vi "Dust_Control_Giraffe_small.vi"(7 "error in":errorcluster) -> (0 "error out":errorcluster)   [LabVIEW 2013]
doc: "This VI specifies the properties of the pulse used for running the dust source. When program is stopped, the voltage is incrementally reduced to zero to avoid quick drops."
uses:
  <vilib>/Utility/miscctls.llb/LVPointTypeDef.ctl
  Functional Global Variables/Action Items.ctl
  <vilib>/Utility/error.llb/DialogType.ctl
  <vilib>/DAQmx/read.llb/DAQmx Read (Analog 1D Wfm NChan NSamp).vi
  <vilib>/Analysis/baseanly.llb/Mean (DBL).vi
  <vilib>/DAQmx/write.llb/DAQmx Write (Analog 1D Wfm NChan NSamp).vi
  <vilib>/DAQmx/read.llb/DAQmx Read (Counter U32 1Chan 1Samp).vi
  <vilib>/addons/database/Connection.llb/Conn Execute.vi
  <vilib>/addons/database/Recordset.llb/Rec Fetch Recordset Data (R).vi
  <vilib>/addons/database/Recordset.llb/Rec Destroy - Connection.vi
  <vilib>/DAQmx/create/channels.llb/DAQmx Create Channel (AI-Voltage-Basic).vi
  <vilib>/DAQmx/configure/timing.llb/DAQmx Timing (Sample Clock).vi
  <vilib>/DAQmx/create/channels.llb/DAQmx Create Channel (AO-Voltage-Basic).vi
  <vilib>/DAQmx/create/channels.llb/DAQmx Create Channel (CI-Count Edges).vi
  <userlib>/_OpenG.lib/comparison/comparison.llb/DBL Changed__ogtk.vi
  <vilib>/measure/mascope.llb/Amplitude and Levels 1 chan.vi
  <vilib>/DAQmx/miscellaneous.llb/DAQmx Fill In Error Info.vi
  Private/throttle.vi
  <userlib>/_OpenG.lib/comparison/comparison.llb/Boolean Changed__ogtk.vi
  Private/throttle from query.vi
  <vilib>/addons/database/_DB Variant To Data/Database Variant To Data.xnode
  <resource>/objmgr/daqmx.rc
  <vilib>/measure/NI_MAPro.lvlib
  <vilib>/Analysis/NI_AALBase.lvlib
  <vilib>/addons/database/NI_Database_API.lvlib
panel:
  out "Freq. Before Throttle":dbl
  out "On/Off":bool
  out "Finished":bool=TRUE
  out "Output waveform":waveform(dbl)={"t0"=timestamp(0 s since 1904-01-01), "dt"=4e-06, "Y"=array[50000 elements]}
  out "Input waveform":waveform(dbl)={"t0"=timestamp(3437998856.0330505 s since 1904-01-01), "dt"=0.00019999999999999998, "Y"=array[1000 elements], "attributes"=variant("NI_ChannelName"=variant(string "Dev5/ai20"), "NI_UnitDescription"=variant(string "Volts"))}
  out "output cluster":T1={"Integer Timestamp"=0, "Needle Voltage"=0.0, "Frequency"=1.0, "Width (ms) : 0.1 "=0.1, "Desired Amplitude (V)"=0.0, "Settings ID"="", "ID#"=0} {"Needle Voltage" min=0.0 max=10.0 step=0.01 format="%.2g"; "Desired Amplitude (V)" min=0.0 max=10.0 step=0.01 format="%5.2f"; "Width (ms) : 0.1" min=0.05 max=5.0 step=0.01 format="%6.2f"; "Frequency" min=1.0 max=100.0 step=0.01 format="%.1f"}
  in  "Tab Control":enum32{"Controls", "Status", "Counter"}(tab)
  in  "Big Accelerator\nSetting?":bool
  out "Actual output width (ms)":dbl caption="Actual Output Width (ms)" format="%.2f"
  out "Actual output Frequency":dbl caption="Actual Output  Frequency (hz)" format="%.2f"
  in  "Width (ms) : 0.1":dbl=0.1 min=0.0 max=5.0 step=0.01 format="%6.2f"
  out "Actual Amplitude (V) 2":dbl=0.0012999050305587314 caption="Actual Amplitude (V)" format="%.2f"
  in  "Desired Amplitude (V)":dbl min=0.0 max=10.0 step=0.01 format="%5.2f"
  out "Actual output Amplitude (V)":dbl caption="Actual Output Amplitude (V)" format="%.2f"
  in  "Frequency":dbl=1.0 caption="Frequency (Hz) : 1" min=0.0 max=30.0 step=0.01 format="%.1f"
  in  "Abort Change":bool
  out "Actual Needle (kV)":dbl=-1.1093266413053247 caption="Actual Einzel (V)" format="%.2f"
  out "Actual Needle Output (V)":dbl caption="Actual Einzel (V)" format="%.2f"
  in  "Needle Voltage":dbl min=0.0 max=10.0 step=0.01 format="%.2g"
  in  "Save Settings?":bool
  out "CONTROLS":waveform(dbl)[](graph)=[{"t0"=timestamp(0 s since 1904-01-01), "dt"=4e-06, "Y"=array[50000 elements]}, {"t0"=timestamp(3437998856.0330505 s since 1904-01-01), "dt"=0.00019999999999999998, "Y"=array[1000 elements], "attributes"=variant("NI_ChannelName"=variant(string "Dev5/ai20"), "NI_UnitDescription"=variant(string "Volts"))}]
  in  "Settings ID":string
  in  "Retrieve Settings":bool
  out "Ratio of particles at\nsecond detector to first":dbl
  out "First detector since\nlast source change:":i64
  out "Average Rate of first":dbl
  out "Average Rate of second":dbl
  in  "# of Cycles ot Average":i32=10
  out "Number of Hours":dbl
  out "Chamber Pressure":dbl format="%#_3g"
  in  "Physical Channels":tag="Dev4/ao0:1" caption="Physical Output Channels"
  in  "Physical Input Channels":tag="Dev6/ai0:2"
  out "Execution Number:":i32=341
  out "Testing":bool
  in  "Counters On/Off":bool=TRUE
  in  "Reset Counters":bool
  in  "Det1":tag="Dev5/ctr0"
  in  "Det2":tag="Dev5/ctr1"
  out "Det2":u32
  out "Det1":u32
  out "error?":bool
  out "Actual Sample Clock Rate":dbl=250000.0 format="%.2f"
  in  "stop":bool
  # "CCLDAS Dust Control Small Accelerator"
  # "Hold Down to\nStop Changes"
  # "Tube Drive (Ao0, Ai4)"
  # "Needle Control (Ao4, Ai0)"
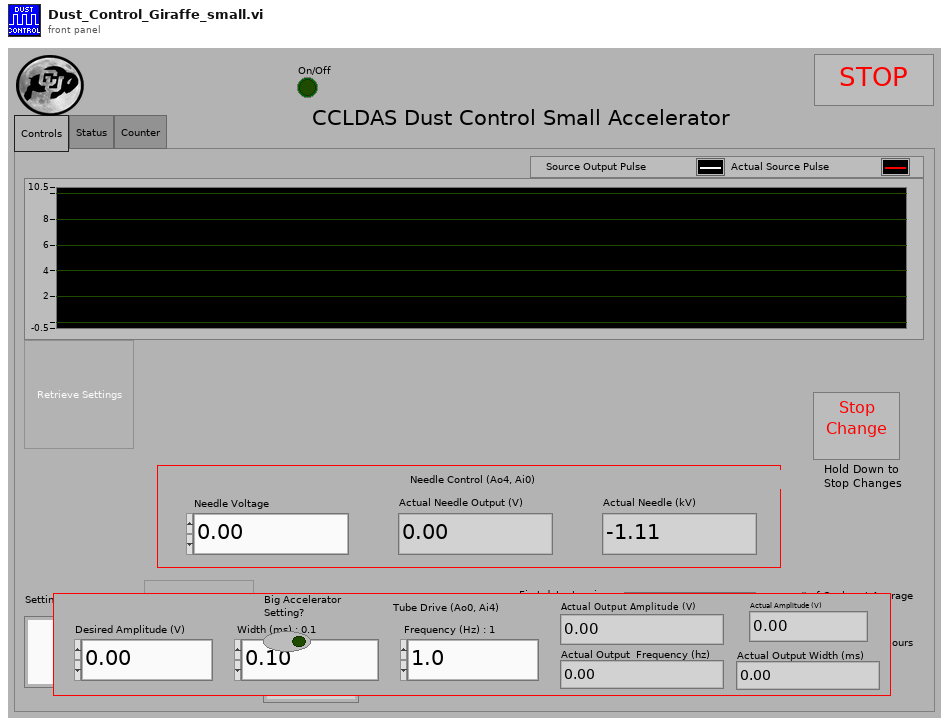
[diagram p1: front panel]
types:
  T1 = cluster{"Integer Timestamp":u64, "Needle Voltage":dbl, "Frequency":dbl, "Width (ms) : 0.1 ":dbl, "Desired Amplitude (V)":dbl, "Settings ID":string, "ID#":i32}
  T2 = typedef "Action Items.ctl" = enum16{"Initialize", "Get", "Set"}
  T3 = typedef "LVPointTypeDef.ctl" = cluster{"Horizontal":i16, "Vertical":i16}
  T4 = typedef "NI_Database_API.lvlib/Conn ObjectReference.ctl" = refnum<k1>
  T5 = typedef "NI_Database_API.lvlib/Rec ObjectReference.ctl" = refnum<k1>
  T6 = enum8{"Enabled", "Disabled", "Disabled and Grayed Out"}
  T7 = typedef "DialogType.ctl" = u16
  T8 = cluster{"Integer Time":i64, "Integer Time":i64, "data":i32}
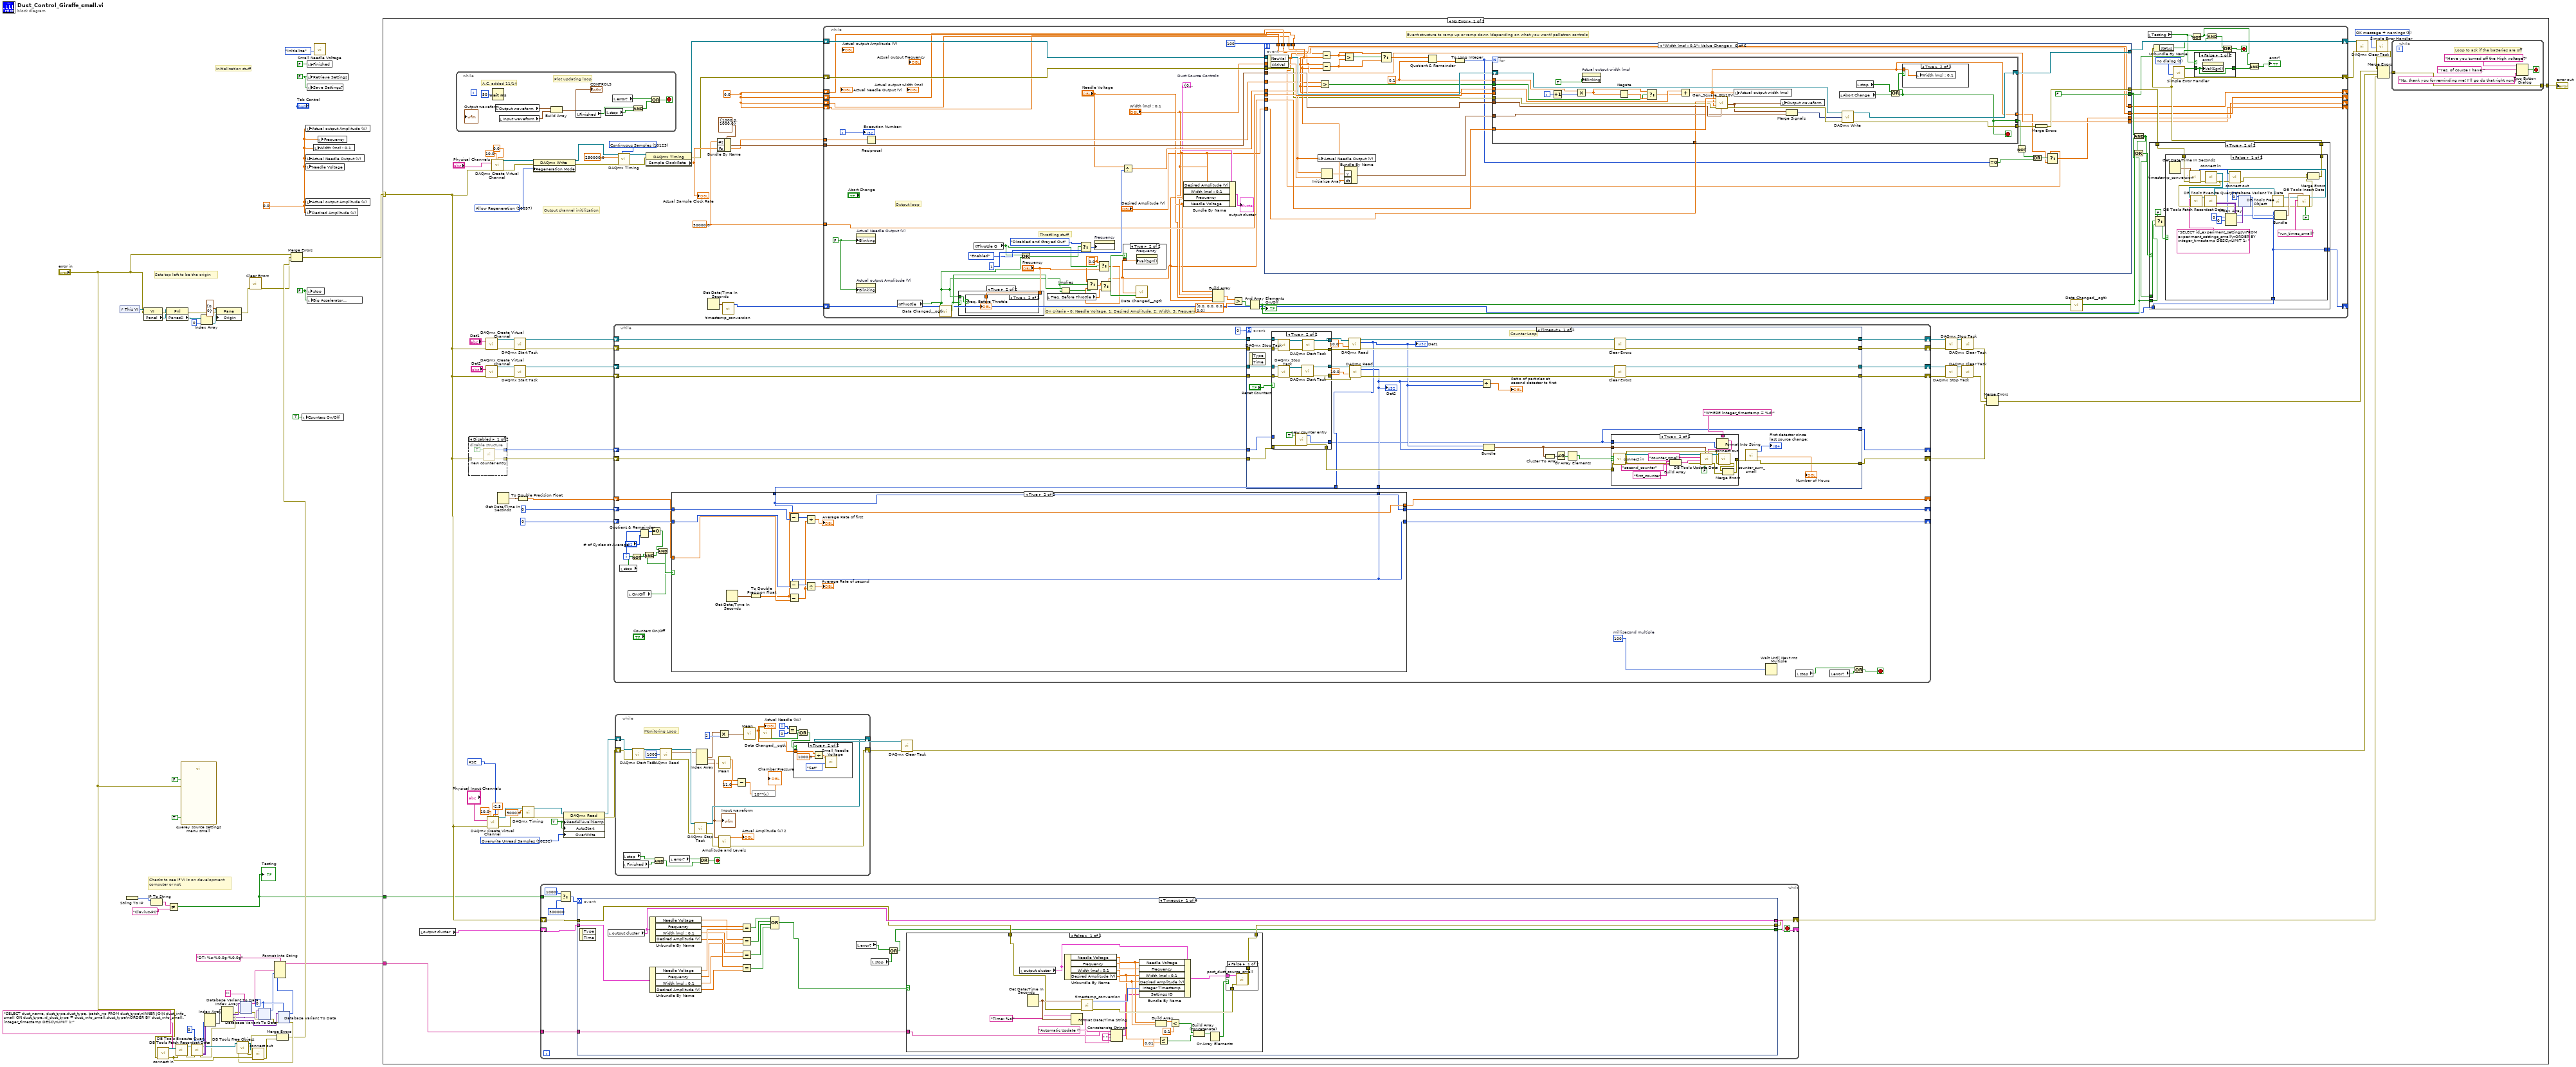
[diagram p0: block diagram]
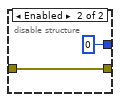
[diagram p2: hidden frame]
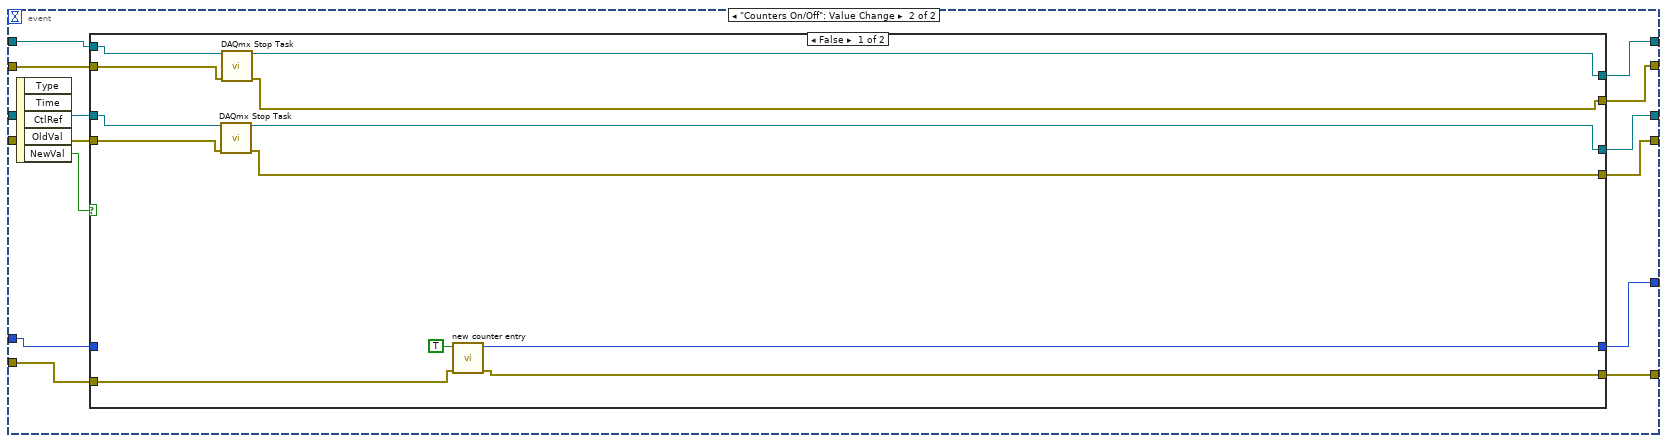
[diagram p5: hidden frame]
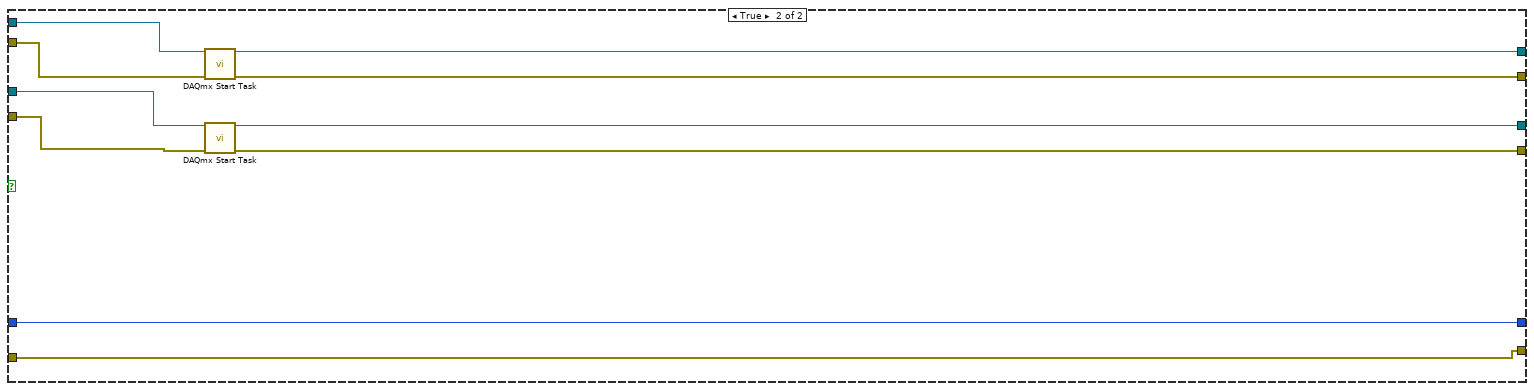
[diagram p6: hidden frame]
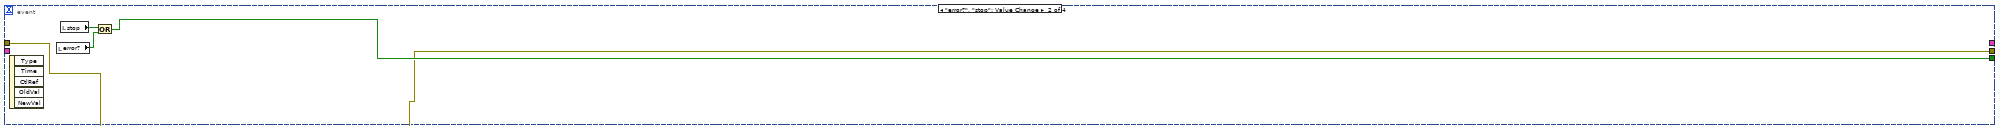
[diagram p11: hidden frame]
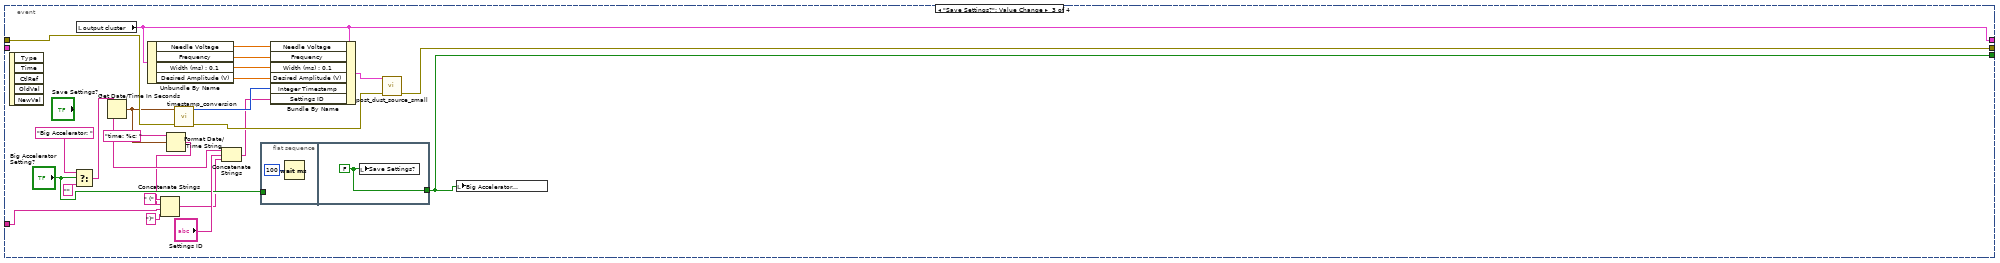
[diagram p12: hidden frame]
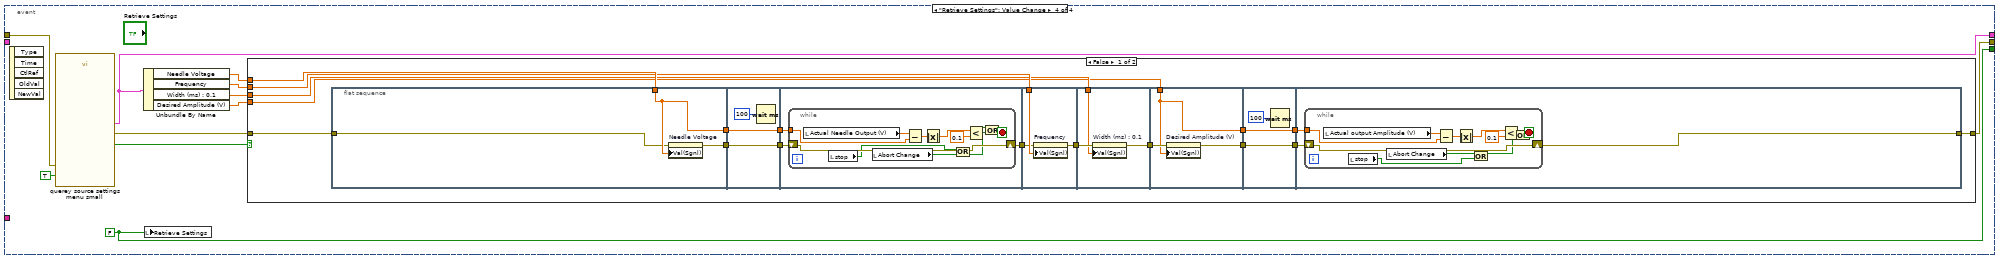
[diagram p13: hidden frame]
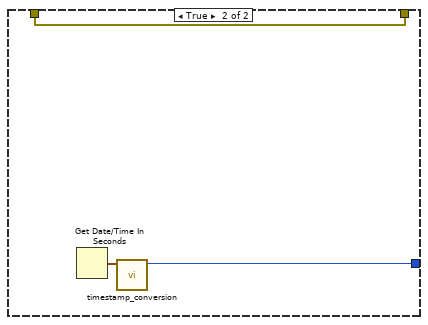
[diagram p19: hidden frame]
diagram:
  w15 = 0
  w50 = FALSE ("Retrieve Settings")
  w48 = 0.0 ("Actual Output (V)")
  w47 = FALSE ("Shutdown")
  # "Checks to see if VI is on development\ncomputer or not"
  # "Sets top left to be the origin"
  # "Initialization stuff"
  n1 = control-ref of="This VI"() -> (w46:refnum<vi>)
  n2 = String To IP() -> (0:w38:u32)  [unwired: 1 in]
  n3 = property class="VI"(reference=w46, error in="error in") -> (error out=w45:errorcluster, "Panel"=w44:refnum<vi>)  [unwired: 1 out]
  n4 = IP To String(2:w38) -> (0:w37:string)  [unwired: 1 in]
  n5 = call "connect in.vi"("error in (no error)"="error in") -> ("error out"=w32:errorcluster, "Database Connection"=w35:T4)  [unwired: 6 in, 1 out]
  n6 = property class="Pnl"(reference=w44, error in=w45) -> (error out=w43:errorcluster, "Panes[]"=w42:refnum<vi>[])  [unwired: 1 out]
  n7 = Not Equal?(x=w37, y="Clavius-PC") -> (x != y?=w8:bool)
  "Testing" <- w8
  n8 = call-poly <vilib>:"DB Tools Execute Query.vi"("error in (no error)"=w32, "SQL query"="SELECT dust_name, dust_type.dust_type, batch_no FROM dust_type\nINNER JOIN dust_info_small ON dust_type.id_dust_type = dust_info_small.dust_type\nORDER BY dust_info_small.integer_timestamp DESC\nLIMIT 1;", "connection reference"=w35) -> ("error out"=w34:errorcluster, "recordset reference"=w33:T5)  [unwired: 5 in]
  n9 = call "querey source settings menu small.vi"("Enable"=FALSE, "subvi?"=TRUE, "error in (no error)"="error in") -> ()  [unwired: 13 in, 4 out]
  n10 = call-poly <vilib>:"DB Tools Fetch Recordset Data.vi"("error in (no error)"=w34, "recordset reference"=w33) -> ("error out"=w20:errorcluster, "recordset data"=w30:variant[][], "recordset reference out"=w29:T5)  [unwired: 3 in]
  n11 = Index Array(array=w42, index=0) -> (element=w40:refnum<vi>)
  n12 = Index Array(array=w30, index (row)=0) -> (element=w24:variant[])  [unwired: 1 in]
  n13 = property class="Pane"(reference=w40, error in=w43, "Origin"=T3 {"Horizontal"=0, "Vertical"=0}) -> (error out=w3:errorcluster)  [unwired: 1 out]
  n14 = Index Array(array=w24) -> (element #1=w23:variant, element #2=w18:variant, element #3=w17:variant)  [unwired: 3 in]
  n15 = xnode "Database Variant To Data"("database variant"=w23, "error in (no error)"=w20, "type"="") -> ("data"=w13:string, "error out"=w22:errorcluster)
  n16 = call <vilib>:"Clear Errors.vi"("error in (no error)"=w3) -> ("error out"=w4:errorcluster)  [unwired: 6 in]
  n17 = xnode "Database Variant To Data"("database variant"=w18, "error in (no error)"=w22, "type"=w15) -> ("data"=w12:i32, "error out"=w21:errorcluster)
  n18 = xnode "Database Variant To Data"("database variant"=w17, "error in (no error)"=w21, "type"=w15) -> ("data"=w11:i32, "error out"=w19:errorcluster)
  n19 = call-poly <vilib>:"DB Tools Free Object.vi"("error in (no error)"=w19, "recordset reference"=w29) -> ("error out"=w28:errorcluster, "connection reference"=w25:T4)  [unwired: 8 in]
  n20 = call "connect out.vi"("error in (no error)"=w32, "connection reference"=w25) -> ("error out"=w27:errorcluster)  [unwired: 9 in]
  n21 = Format Into String(format string="DT: %s-%0.0g-%0.0g", w13, w12, w11) -> (resulting string=w9:string)  [unwired: 2 in, 1 out]
  n22 = Merge Errors(w28, w27) -> (w10:errorcluster)
  n23 = Merge Errors("error in", w4, w10) -> (w5:errorcluster)
  n24 = local write "Counters On/Off"(TRUE ("Counters On/Off")) -> ()
  n25 = local write "Actual output Amplitude (V)"(w48) -> ()
  n26 = local write "Actual Needle Output (V)"(w48) -> ()
  n27 = local write "Needle Voltage"(w48) -> ()
  n28 = local write "Actual output Amplitude (V)"(w48) -> ()
  n29 = local write "Desired Amplitude (V)"(w48) -> ()
  n30 = local write "Finished"(FALSE ("Finished")) -> ()
  n31 = local write "Retrieve Settings"(w50) -> ()
  n32 = local write "Save Settings?"(w50) -> ()
  n33 = local write "stop"(w47) -> ()
  n34 = local write "Big Accelerator\nSetting?"(w47) -> ()
  n35 = local write "Width (ms) : 0.1"(w48) -> ()
  n36 = call "Small Needle Voltage.vi"("Action"=Action_Items."Initialize") -> ()  [unwired: 10 in, 1 out]
  n37 = local write "Frequency"(w48) -> ()
  n38 = case shown="No Error" w5 {
    selector: w5 -> [w65 w994]
    tunnel: [w107 w994] -> w52
    tunnel: w9 -> [w55 _]
    tunnel: w8 -> [w54 _]
    frame No Error {
      w53 = 10083 items=["default"=-1, "RSE"=10083, "NRSE"=10078, "Differential"=10106, "Pseudodifferential"=12529] ("input terminal configuration")
      w62 = 0.0 ("Width (ms) : 3.5")
      w75 = 10252 items=["Overwrite Unread Samples"=10252, "Do Not Overwrite Unread Samples"=10159] ("OverWrite")
      w76 = TRUE ("ReadAllAvailSamp")
      w58 = 50000.0 ("Size (Samples)")
      w120 = 10097 items=["Allow Regeneration"=10097, "Do Not Allow Regeneration"=10158] ("RegenMode")
      w125 = T7 3 items=["no dialog", "OK message", "continue or stop message", "OK message + warnings", "continue/stop + warnings"] ("type of dialog (OK msg:1)")
      w129 = 10123 items=["Finite Samples"=10178, "Continuous Samples"=10123] ("sample mode")
      # "Output channel initilization"
      n39 = local read "output cluster"() -> (w57:T1)
      n40 = while {
        stop <- w304 stop-if-true
        # "Plot updating loop"
        # "A.C. added 11/14"
        n41 = Wait (ms)(milliseconds to wait=u32 50) -> ()  [unwired: 1 out]
        n42 = local read "Output waveform"() -> (w301:waveform(dbl))
        n43 = local read "Input waveform"() -> (w302:waveform(dbl))
        n44 = Build Array(w301, w302) -> (→"CONTROLS":waveform(dbl)[])
        n45 = local read "Finished"() -> (w299:bool)
        n46 = local read "stop"() -> (w300:bool)
        n47 = local read "error?"() -> (w303:bool)
        n48 = And(x=w299, y=w300) -> (x .and. y?=w298:bool)
        n49 = Or(x=w303, y=w298) -> (x .or. y?=w304:bool)
      }
      n50 = disable-structure shown="Disabled" {
        disable-tunnel: [w133 w135] -> w84
        disable-tunnel: [w132 i64 0 ("Integer Time")] -> w83
        disable-tunnel: w65 -> [w131 w135]
        frame Disabled {
          n51 = call "new counter entry.vi"("error in"=w131, "Small?"=TRUE) -> ("error out"=w133:errorcluster, "Integer Time"=w132:i64)  [unwired: 8 in]
        }
        frame Enabled {
        }
      }
      n52 = call-poly <vilib>:"DAQmx Create Virtual Channel.vi"("counter"="Det1", "error in"=w65) -> ("task out"=w92:refnum<k21>, "error out"=w89:errorcluster)  [unwired: 12 in]
      n53 = call-poly <vilib>:"DAQmx Create Virtual Channel.vi"("counter"="Det2", "error in"=w65) -> ("task out"=w91:refnum<k21>, "error out"=w90:errorcluster)  [unwired: 12 in]
      n54 = call-poly <vilib>:"DAQmx Create Virtual Channel.vi"("maximum value"=10.0 ("Maximum Value"), "minimum value"=-2.5 ("Minimum Value"), "input terminal configuration"=w53, "physical channels"="Physical Input Channels", "error in"=w65) -> ("task out"=w69:refnum<k21>, "error out"=w68:errorcluster)  [unwired: 9 in]
      n55 = call-poly <vilib>:"DAQmx Create Virtual Channel.vi"("maximum value"=10.0 ("Maximum Value"), "minimum value"=0.0 ("Minimum Value"), "physical channels"="Physical Channels", "error in"=w65) -> ("task out"=w119:refnum<k21>, "error out"=w118:errorcluster)  [unwired: 10 in]
      n56 = Get Date/Time In Seconds() -> (seconds since 1Jan1904=w82:timestamp)
      n57 = call <vilib>:"DAQmx Start Task.vi"("task/channels in"=w92, "error in"=w89) -> ("task out"=w104:refnum<k21>, "error out"=w101:errorcluster)  [unwired: 12 in]
      n58 = call <vilib>:"DAQmx Start Task.vi"("task/channels in"=w91, "error in"=w90) -> ("task out"=w103:refnum<k21>, "error out"=w102:errorcluster)  [unwired: 12 in]
      n59 = To Double Precision Float(number=w82) -> (double precision float=w81:dbl)
      n60 = call-poly <vilib>:"DAQmx Timing.vi"("task/channels in"=w69, "rate"=5000.0, "error in"=w68) -> ("task out"=w74:refnum<k21>, "error out"=w73:errorcluster)  [unwired: 11 in]
      n61 = property class="DAQmx Write"(reference=w119, error in=w118, "Regeneration Mode"=w120) -> (reference out=w117:refnum<k21>, error out=w116:errorcluster)
      n62 = while {
        shift-right: [w349] -> w86
        shift-left: w65 -> [w348]
        shift-right: [w351] -> _
        shift-left: w57 -> [w350]
        tunnel: w54 -> [w344]
        tunnel: w55 -> [w342]
        stop <- w347 stop-if-true
        n63 = Select(t=1000, s=w344, f=300000) -> (s? t:f=w346:i32)
        n64 = event shown="[0] Timeout" {
          selector: _ -> [_ _ _ _]
          dyn-events: _ -> [_ _ _ _]
          timeout: w346 -> [_ _ _ _]
          tunnel: [w372 _ w414 w433] -> w351
          tunnel: w350 -> [w371 _ _ _]
          tunnel: [w356 w402 w429 w436] -> w349
          tunnel: w348 -> [w357 w402 w426 w442]
          tunnel: [w354 w403 w415 w435] -> w347
          tunnel: w342 -> [w358 _ w410 _]
          event Timeout {
            n65 = event-data() -> ()  [unwired: 1 in, 2 out]
            n66 = local read "output cluster"() -> (w372:T1)
            n67 = Unbundle By Name(w372) -> ("Needle Voltage"=w370:dbl, "Frequency"=w368:dbl, "Width (ms) : 0.1"=w366:dbl, "Desired Amplitude (V)"=w364:dbl)
            n68 = Unbundle By Name(w371) -> ("Needle Voltage"=w369:dbl, "Frequency"=w367:dbl, "Width (ms) : 0.1"=w359:dbl, "Desired Amplitude (V)"=w365:dbl)
            n69 = Equal?(x=w370, y=w369) -> (x = y?=w363:bool)
            n70 = Equal?(x=w368, y=w367) -> (x = y?=w362:bool)
            n71 = Equal?(x=w366, y=w359) -> (x = y?=w361:bool)
            n72 = Equal?(x=w364, y=w365) -> (x = y?=w360:bool)
            n73 = Compound Arithmetic op=OR(w363, w362, w361, w360) -> (w355:bool)
            n74 = local read "error?"() -> (w353:bool)
            n75 = local read "stop"() -> (w352:bool)
            n76 = Or(x=w353, y=w352) -> (x .or. y?=w354:bool)
            n77 = case shown="False" w355 {
              tunnel: w358 -> [w373 _]
              tunnel: w357 -> [w378 w401]
              tunnel: [w377 w401] -> w356
              frame False {
                n78 = local read "output cluster"() -> (w382:T1)
                n79 = Get Date/Time In Seconds() -> (seconds since 1Jan1904=w394:timestamp)
                n80 = Unbundle By Name(w382) -> ("Needle Voltage"=w392:dbl, "Frequency"=w388:dbl, "Width (ms) : 0.1"=w387:dbl, "Desired Amplitude (V)"=w391:dbl)
                n81 = Format Date/Time String(time format string (%c)="Time: %c)" ("Settings ID"), seconds (now)=w394) -> (date/time string=w374:string)  [unwired: 1 in]
                n82 = call "timestamp_conversion.vi"("error in (no error)"=w378, "Time Stamp"=w394) -> ("error out"=w395:errorcluster, "Integer Time"=w396:i64)  [unwired: 7 in]
                n83 = Concatenate Strings("Automatic Update (" ("string"), w373, " " ("string"), w374) -> (w380:string)
                n84 = Bundle By Name(cluster=w382, "Needle Voltage"=w392, "Frequency"=w388, "Width (ms) : 0.1"=w387, "Desired Amplitude (V)"=w391, "Integer Timestamp"=w396, "Settings ID"=w380) -> (w383:T1)
                n85 = Build Array(w392, w391) -> (w390:dbl[])
                n86 = Less Or Equal?(x=w387, y=0.01) -> (x <= y?=w381:bool)
                n87 = Less?(x=w390, y=0.1) -> (x < y?=w385:bool[])
                n88 = Build Array (concatenate)(w385, w381) -> (w384:bool[])
                n89 = Or Array Elements(Boolean array=w384) -> (logical OR=w379:bool)
                n90 = case shown="False" w379 {
                  tunnel: w383 -> [w397 _]
                  tunnel: [w399 w400] -> w377
                  tunnel: w395 -> [w398 w400]
                  frame False {
                    n91 = call "post_dust_source_small.vi"("error in (no error)"=w398, "Dust control settings"=w397) -> ("error out"=w399:errorcluster)  [unwired: 8 in, 1 out]
                  }
                  frame True {
                  }
                }
              }
              frame True {
              }
            }
          }
          event "error?", "stop": Value Change {
            n92 = event-data() -> ()  [unwired: 1 in, 5 out]
            n93 = local read "error?"() -> (w404:bool)
            n94 = local read "stop"() -> (w405:bool)
            n95 = Or(x=w405, y=w404) -> (x .or. y?=w403:bool)
          }
          event "Save Settings?": Value Change {
            n96 = event-data() -> ()  [unwired: 1 in, 5 out]
            n97 = Select(t="Big Accelerator: ", s="Big Accelerator\nSetting?", f="") -> (s? t:f=w417:string)
            n98 = local read "output cluster"() -> (w414:T1)
            n99 = Get Date/Time In Seconds() -> (seconds since 1Jan1904=w424:timestamp)
            n100 = Unbundle By Name(w414) -> ("Needle Voltage"=w423:dbl, "Frequency"=w422:dbl, "Width (ms) : 0.1"=w421:dbl, "Desired Amplitude (V)"=w420:dbl)
            n101 = Format Date/Time String(time format string (%c)="time: %c; " ("Settings ID"), seconds (now)=w424) -> (date/time string=w408:string)  [unwired: 1 in]
            n102 = Concatenate Strings(" (" ("string"), w408, w410, ")" ("string")) -> (w407:string)
            n103 = call "timestamp_conversion.vi"("error in (no error)"=w426, "Time Stamp"=w424) -> ("error out"=w427:errorcluster, "Integer Time"=w428:i64)  [unwired: 7 in]
            n104 = Concatenate Strings(w417, "Settings ID", w407) -> (w406:string)
            n105 = flat-sequence {
              tunnel: "Big Accelerator\nSetting?" -> [_]
              tunnel: [w431] -> w415
              frame #0 {
                n106 = Wait (ms)(milliseconds to wait=u32 100) -> ()  [unwired: 1 out]
              }
              frame #1 {
                w431 = FALSE
                n107 = local write "Save Settings?"(w431) -> ()
              }
            }
            n108 = Bundle By Name(cluster=w414, "Needle Voltage"=w423, "Frequency"=w422, "Width (ms) : 0.1"=w421, "Desired Amplitude (V)"=w420, "Integer Timestamp"=w428, "Settings ID"=w406) -> (w413:T1)
            n109 = call "post_dust_source_small.vi"("error in (no error)"=w427, "Dust control settings"=w413) -> ("error out"=w429:errorcluster)  [unwired: 8 in, 1 out]
            n110 = local write "Big Accelerator\nSetting?"(w415) -> ()
          }
          event "Retrieve Settings": Value Change {
            w435 = FALSE
            n111 = event-data() -> ()  [unwired: 1 in, 5 out]
            n112 = call "querey source settings menu small.vi"("subvi?"=TRUE, "error in (no error)"=w442) -> ("Output cluster"=w433:T1, "Cancel loading"=w434:bool, "error out"=w441:errorcluster)  [unwired: 14 in, 1 out]
            n113 = Unbundle By Name(w433) -> ("Needle Voltage"=w440:dbl, "Frequency"=w439:dbl, "Width (ms) : 0.1"=w438:dbl, "Desired Amplitude (V)"=w437:dbl)
            n114 = local write "Retrieve Settings"(w435) -> ()
            n115 = case shown="False" w434 {
              tunnel: w441 -> [w459 w506]
              tunnel: w440 -> [w458 _]
              tunnel: w439 -> [w457 _]
              tunnel: w438 -> [w455 _]
              tunnel: w437 -> [w446 _]
              tunnel: [w443 w506] -> w436
              frame False {
                n116 = flat-sequence {
                  tunnel: w458 -> [w461]
                  tunnel: [w462] -> w454
                  tunnel: [w461] -> w450
                  tunnel: w459 -> [w460]
                  tunnel: w454 -> [w465]
                  tunnel: [w465] -> w453
                  tunnel: [w463] -> w451
                  tunnel: w450 -> [w463]
                  tunnel: w453 -> [w467]
                  tunnel: w451 -> [w468]
                  tunnel: [w466] -> w449
                  tunnel: w457 -> [w482]
                  tunnel: [w481] -> w456
                  tunnel: w449 -> [w480]
                  tunnel: w456 -> [w485]
                  tunnel: w455 -> [w483]
                  tunnel: [w484] -> w448
                  tunnel: w448 -> [w488]
                  tunnel: [w486] -> w447
                  tunnel: w446 -> [w487]
                  tunnel: [w487] -> w445
                  tunnel: w447 -> [w491]
                  tunnel: [w491] -> w452
                  tunnel: w445 -> [w489]
                  tunnel: [w489] -> w444
                  tunnel: [w494] -> w443
                  tunnel: w452 -> [w493]
                  tunnel: w444 -> [w492]
                  frame #0 {
                    n117 = property on="Needle Voltage" class="DigNum (strict)"(error in=w460, "Val(Sgnl)"=w461) -> (error out=w462:errorcluster)  [unwired: 1 in, 1 out]
                  }
                  frame #1 {
                    n118 = Wait (ms)(milliseconds to wait=u32 100) -> ()  [unwired: 1 out]
                  }
                  frame #2 {
                    n119 = while {
                      tunnel: w468 -> [w474]
                      shift-right: [w479] -> w466
                      shift-left: w467 -> [w479]
                      stop <- w472 stop-if-true
                      n120 = local read "Actual Needle Output (V)"() -> (w475:dbl)
                      n121 = local read "stop"() -> (w469:bool)
                      n122 = local read "Abort Change"() -> (w471:bool)
                      n123 = Subtract(x=w475, y=w474) -> (x-y=w478:dbl)
                      n124 = Absolute Value(x=w478) -> (abs(x)=w477:dbl)
                      n125 = Or(x=w469, y=w471) -> (x .or. y?=w470:bool)
                      n126 = Less?(x=w477, y=0.1) -> (x < y?=w473:bool)
                      n127 = Or(x=w470, y=w473) -> (x .or. y?=w472:bool)
                    }
                  }
                  frame #3 {
                    n128 = property on="Frequency" class="DigNum (strict)"(error in=w480, "Val(Sgnl)"=w482) -> (error out=w481:errorcluster)  [unwired: 1 in, 1 out]
                  }
                  frame #4 {
                    n129 = property on="Width (ms) : 0.1" class="DigNum (strict)"(error in=w485, "Val(Sgnl)"=w483) -> (error out=w484:errorcluster)  [unwired: 1 in, 1 out]
                  }
                  frame #5 {
                    n130 = property on="Desired Amplitude (V)" class="DigNum (strict)"(error in=w488, "Val(Sgnl)"=w487) -> (error out=w486:errorcluster)  [unwired: 1 in, 1 out]
                  }
                  frame #6 {
                    n131 = Wait (ms)(milliseconds to wait=u32 100) -> ()  [unwired: 1 out]
                  }
                  frame #7 {
                    n132 = while {
                      tunnel: w492 -> [w505]
                      shift-right: [w503] -> w494
                      shift-left: w493 -> [w503]
                      stop <- w498 stop-if-true
                      n133 = local read "Actual output Amplitude (V)"() -> (w504:dbl)
                      n134 = local read "stop"() -> (w495:bool)
                      n135 = local read "Abort Change"() -> (w496:bool)
                      n136 = Subtract(x=w504, y=w505) -> (x-y=w501:dbl)
                      n137 = Absolute Value(x=w501) -> (abs(x)=w500:dbl)
                      n138 = Or(x=w496, y=w495) -> (x .or. y?=w497:bool)
                      n139 = Less?(x=w500, y=0.1) -> (x < y?=w502:bool)
                      n140 = Or(x=w502, y=w497) -> (x .or. y?=w498:bool)
                    }
                  }
                }
              }
              frame True {
              }
            }
          }
        }
      }
      n141 = property class="DAQmx Read"(reference=w74, error in=w73, "ReadAllAvailSamp"=w76, "AutoStart"=w76, "OverWrite"=w75) -> (reference out=w66:refnum<k21>, error out=w64:errorcluster)
      n142 = while {
        shift-right: [w155] -> _
        shift-left: w83 -> [w157]
        shift-right: [w150] -> _
        shift-left: w81 -> [w146]
        shift-right: [w149] -> _
        shift-left: u32 0 ("data") -> [w153]
        shift-right: [w148] -> _
        shift-left: u32 0 ("data") -> [w152]
        shift-right: [w169] -> w100
        shift-left: w104 -> [w161]
        shift-right: [w163] -> w99
        shift-left: w101 -> [w160]
        shift-right: [w168] -> w98
        shift-left: w103 -> [w159]
        shift-right: [w167] -> w97
        shift-left: w102 -> [w158]
        shift-right: [w162] -> w59
        shift-left: w84 -> [w156]
        i -> [w138]
        stop <- w164 stop-if-true
        w166 = u32 100  # millisecond multiple
        n143 = local read "stop"() -> (w145:bool)
        n144 = local read "On/Off"() -> (w137:bool)
        n145 = Not(x=w145) -> (.not. x?=w144:bool)
        n146 = Quotient & Remainder(x=w138, y="# of Cycles ot Average") -> (x-y*floor(x/y)=w147:i32)  [unwired: 1 out]
        n147 = And(x=w144, y=w137) -> (x .and. y?=w141:bool)
        n148 = Equal To 0?(x=w147) -> (x = 0?=w142:bool)
        n149 = And(x=w142, y=w141) -> (x .and. y?=w143:bool)
        n150 = event shown="[0] Timeout" {
          selector: _ -> [_ _]
          dyn-events: _ -> [_ _]
          timeout: 0 -> [_ _]
          tunnel: [w202 w251] -> w169
          tunnel: [w199 w249] -> w168
          tunnel: [w198 w248] -> w167
          tunnel: [w194 w250] -> w163
          tunnel: [w193 w242] -> w162
          tunnel: w161 -> [w190 w246]
          tunnel: w160 -> [w189 w253]
          tunnel: w159 -> [w188 w247]
          tunnel: w158 -> [w187 w252]
          tunnel: w157 -> [w181 w245]
          tunnel: w156 -> [w180 w243]
          tunnel: [w171 w244] -> w155
          tunnel: [w177 _] -> w151
          tunnel: [w172 _] -> w136
          event Timeout {
            # "Counter Loop"
            n151 = event-data() -> ()  [unwired: 1 in, 2 out]
            n152 = case shown="True" "Reset Counters" {
              tunnel: w190 -> [w225 w241]
              tunnel: [w225 w239] -> w186
              tunnel: w189 -> [w224 w238]
              tunnel: [w224 w236] -> w185
              tunnel: w188 -> [w223 w235]
              tunnel: [w223 w233] -> w184
              tunnel: w187 -> [w222 w232]
              tunnel: [w222 w230] -> w183
              tunnel: w180 -> [w221 w228]
              tunnel: [w220 w229] -> w171
              tunnel: [w221 w227] -> w179
              tunnel: w181 -> [w220 _]
              frame False {
              }
              frame True {
                n153 = call <vilib>:"DAQmx Stop Task.vi"("task/channels in"=w235, "error in"=w232) -> ("task out"=w234:refnum<k21>, "error out"=w231:errorcluster)  [unwired: 12 in]
                n154 = call <vilib>:"DAQmx Stop Task.vi"("task/channels in"=w241, "error in"=w238) -> ("task out"=w240:refnum<k21>, "error out"=w237:errorcluster)  [unwired: 12 in]
                n155 = call "new counter entry.vi"("error in"=w228, "Small?"=TRUE) -> ("error out"=w227:errorcluster, "Integer Time"=w229:i64)  [unwired: 8 in]
                n156 = call <vilib>:"DAQmx Start Task.vi"("task/channels in"=w234, "error in"=w231) -> ("task out"=w233:refnum<k21>, "error out"=w230:errorcluster)  [unwired: 12 in]
                n157 = call <vilib>:"DAQmx Start Task.vi"("task/channels in"=w240, "error in"=w237) -> ("task out"=w239:refnum<k21>, "error out"=w236:errorcluster)  [unwired: 12 in]
              }
            }
            n158 = call-poly <vilib>:"DAQmx Read.vi"("task/channels in"=w186, "timeout"=10.0, "error in"=w185) -> ("task out"=w202:refnum<k21>, "data"=w177:u32, "error out"=w197:errorcluster)  [unwired: 10 in]
            "Det1" <- w177
            n159 = call-poly <vilib>:"DAQmx Read.vi"("task/channels in"=w184, "timeout"=10.0, "error in"=w183) -> ("task out"=w199:refnum<k21>, "data"=w172:u32, "error out"=w196:errorcluster)  [unwired: 10 in]
            "Det2" <- w172
            n160 = Divide(x=w172, y=w177) -> (x/y=→"Ratio of particles at\nsecond detector to first":dbl)
            n161 = Bundle("data"=w177, "data"=w172) -> (w170:cluster{"data":u32, "data":u32})  [unwired: 1 in]
            n162 = Cluster To Array(cluster=w170) -> (array=w176:u32[])
            n163 = Not Equal To 0?(x=w176) -> (x != 0?=w175:bool[])
            n164 = Or Array Elements(Boolean array=w175) -> (logical OR=w174:bool)
            n165 = case shown="True" w174 {
              tunnel: [w203 w209] -> w192
              tunnel: "WHERE integer_timestamp = %d;" ("condition") -> [_ w208]
              tunnel: w179 -> [w203 w206]
              tunnel: w171 -> [_ w205]
              tunnel: w170 -> [_ w204]
              frame False {
              }
              frame True {
                n166 = call "connect in.vi"("error in (no error)"=w206) -> ("error out"=w212:errorcluster, "Database Connection"=w218:T4)  [unwired: 6 in, 1 out]
                n167 = Build Array("first_counter" ("string"), "second_counter" ("string")) -> (w214:string[])
                n168 = Format Into String(format string=w208, w205) -> (resulting string=w207:string)  [unwired: 2 in, 1 out]
                n169 = call <vilib>:"DB Tools Update Data.vi"("condition"=w207, "flatten cluster? (F)"=FALSE ("create table? (F)"), "data"=w204, "error in (no error)"=w212, "columns"=w214, "table"="counter_small", "connection reference"=w218) -> ("error out"=w210:errorcluster, "connection reference out"=w216:T4)  [unwired: 3 in]
                n170 = call "connect out.vi"("error in (no error)"=w212, "connection reference"=w216) -> ("error out"=w211:errorcluster)  [unwired: 9 in]
                n171 = Merge Errors(w211, w210) -> (w209:errorcluster)
              }
            }
            n172 = call <vilib>:"Clear Errors.vi"("error in (no error)"=w197) -> ("error out"=w194:errorcluster)  [unwired: 6 in]
            n173 = call <vilib>:"Clear Errors.vi"("error in (no error)"=w196) -> ("error out"=w198:errorcluster)  [unwired: 6 in]
            n174 = call "counter_sum_small.vi"("error in"=w192) -> ("error IO"=w193:errorcluster, "Number of Hours"=→"Number of Hours":dbl, "First Detector Sum"=→"First detector since\nlast source change:":i64)  [unwired: 7 in, 1 out]
          }
          event "Counters On/Off": Value Change {
            n175 = event-data() -> ("NewVal"=w254:bool)  [unwired: 1 in, 4 out]
            n176 = case shown="False" w254 {
              tunnel: w253 -> [w265 w272]
              tunnel: w252 -> [w263 w271]
              tunnel: [w259 w276] -> w251
              tunnel: [w260 w275] -> w250
              tunnel: [w261 w274] -> w249
              tunnel: [w262 w273] -> w248
              tunnel: w247 -> [w264 w270]
              tunnel: w246 -> [w266 w269]
              tunnel: w245 -> [_ w268]
              tunnel: [w258 w268] -> w244
              tunnel: w243 -> [w257 w267]
              tunnel: [w256 w267] -> w242
              frame False {
                n177 = call <vilib>:"DAQmx Stop Task.vi"("task/channels in"=w264, "error in"=w263) -> ("task out"=w261:refnum<k21>, "error out"=w262:errorcluster)  [unwired: 12 in]
                n178 = call <vilib>:"DAQmx Stop Task.vi"("task/channels in"=w266, "error in"=w265) -> ("task out"=w259:refnum<k21>, "error out"=w260:errorcluster)  [unwired: 12 in]
                n179 = call "new counter entry.vi"("error in"=w257, "Small?"=TRUE) -> ("error out"=w256:errorcluster, "Integer Time"=w258:i64)  [unwired: 8 in]
              }
              frame True {
                n180 = call <vilib>:"DAQmx Start Task.vi"("task/channels in"=w269, "error in"=w272) -> ("task out"=w276:refnum<k21>, "error out"=w275:errorcluster)  [unwired: 12 in]
                n181 = call <vilib>:"DAQmx Start Task.vi"("task/channels in"=w270, "error in"=w271) -> ("task out"=w274:refnum<k21>, "error out"=w273:errorcluster)  [unwired: 12 in]
              }
            }
          }
        }
        n182 = case shown="True" w143 {
          tunnel: w146 -> [w279 w290]
          tunnel: w153 -> [w278 w289]
          tunnel: w152 -> [w277 w288]
          tunnel: w151 -> [_ w283]
          tunnel: [w279 w284] -> w150
          tunnel: [w278 w283] -> w149
          tunnel: [w277 w280] -> w148
          tunnel: w136 -> [_ w280]
          frame False {
          }
          frame True {
            n183 = Get Date/Time In Seconds() -> (seconds since 1Jan1904=w291:timestamp)
            n184 = To Double Precision Float(number=w291) -> (double precision float=w284:dbl)
            n185 = Subtract(x=w283, y=w289) -> (x-y=w287:u32)
            n186 = Subtract(x=w280, y=w288) -> (x-y=w286:u32)
            n187 = Subtract(x=w284, y=w290) -> (x-y=w285:dbl)
            n188 = Divide(x=w287, y=w285) -> (x/y=→"Average Rate of first":dbl)
            n189 = Divide(x=w286, y=w285) -> (x/y=→"Average Rate of second":dbl)
          }
        }
        n190 = Wait Until Next ms Multiple(millisecond multiple=w166) -> ()  [unwired: 1 out]
        n191 = local read "stop"() -> (w139:bool)
        n192 = local read "error?"() -> (w165:bool)
        n193 = Or(x=w139, y=w165) -> (x .or. y?=w164:bool)
      }
      n194 = while {
        shift-right: [w318] -> w63
        shift-left: w66 -> [w320]
        shift-right: [w321] -> w78
        shift-left: w64 -> [w319]
        i -> [w308]
        stop <- w322 stop-if-true
        # "Monitoring Loop"
        n195 = local read "stop"() -> (w336:bool)
        n196 = local read "Finished"() -> (w337:bool)
        n197 = call <vilib>:"DAQmx Start Task.vi"("task/channels in"=w320, "error in"=w319) -> ("task out"=w327:refnum<k21>, "error out"=w328:errorcluster)  [unwired: 12 in]
        n198 = And(x=w336, y=w337) -> (x .and. y?=w335:bool)
        n199 = call-poly <vilib>:"DAQmx Read.vi"("task/channels in"=w327, "number of samples per channel"=1000, "error in"=w328) -> ("task out"=w329:refnum<k21>, "data"=w323:waveform(dbl)[], "error out"=w330:errorcluster)  [unwired: 10 in]
        n200 = local read "error?"() -> (w324:bool)
        n201 = call <vilib>:"DAQmx Stop Task.vi"("task/channels in"=w329, "error in"=w330) -> ("task out"=w318:refnum<k21>, "error out"=w334:errorcluster)  [unwired: 12 in]
        n202 = Index Array(array=w323) -> (element #1=w325:waveform(dbl), element #2=w317:waveform(dbl), element #3=w316:waveform(dbl))  [unwired: 3 in]
        "Input waveform" <- w317
        n203 = Or(x=w324, y=w335) -> (x .or. y?=w322:bool)
        n204 = Multiply(x=w325, y=2) -> (x*y=w331:waveform(dbl))
        n205 = call-poly <vilib>:"Mean.vi"("X"=w316) -> ("mean"=w315:dbl)  [unwired: 1 out]
        n206 = call-poly <vilib>:"Amplitude and Levels.vi"("error in (no error)"=w334, "signal in"=w317) -> ("error out"=w321:errorcluster, "amplitude"=→"Actual Amplitude (V) 2":dbl)  [unwired: 6 in, 2 out]
        n207 = Subtract(x=w315, y=11.0) -> (x-y=w313:dbl)
        n208 = call-poly <vilib>:"Mean.vi"("X"=w331) -> ("mean"=w311:dbl)  [unwired: 1 out]
        "Actual Needle (kV)" <- w311
        n209 = expression code="10**(x)"(w313) -> (→"Chamber Pressure":dbl)
        n210 = call-poly <userlib>:"Data Changed__ogtk.vi"("DBL"=w311) -> ("Changed"=w309:bool)
        n211 = Equal?(x=w308, y=0) -> (x = y?=w306:bool)
        n212 = Or(x=w306, y=w309) -> (x .or. y?=w310:bool)
        n213 = case shown="True" w310 {
          tunnel: w311 -> [_ w339]
          frame False {
          }
          frame True {
            n214 = Divide(x=w339, y=1000.0) -> (x/y=w340:dbl)
            n215 = call "Small Needle Voltage.vi"("Action"=Action_Items."Set", "Input Pelletron Voltage"=w340) -> ()  [unwired: 9 in, 1 out]
          }
        }
      }
      n216 = call-poly <vilib>:"DAQmx Timing.vi"("task/channels in"=w117, "sample mode"=w129, "rate"=250000.0 ("Sample Clock Rate"), "error in"=w116) -> ("task out"=w123:refnum<k21>, "error out"=w109:errorcluster)  [unwired: 10 in]
      n217 = property class="DAQmx Timing"(reference=w123, error in=w109) -> (reference out=w111:refnum<k21>, error out=w56:errorcluster, "Sample Clock:Rate"=w115:dbl)
      "Actual Sample Clock Rate" <- w115
      n218 = Get Date/Time In Seconds() -> (seconds since 1Jan1904=w61:timestamp)
      n219 = Bundle By Name(cluster=cluster{"Fs":dbl, "#s":dbl} {"Fs"=1000.0, "#s"=1000.0} ("sampling info"), "#s"=w58, "Fs"=w115) -> (w121:cluster{"Fs":dbl, "#s":dbl})
      n220 = call "timestamp_conversion.vi"("Time Stamp"=w61) -> ("Integer Time"=w60:i64)  [unwired: 8 in, 1 out]
      n221 = while {
        tunnel: w121 -> [w566]
        tunnel: w115 -> [w564]
        tunnel: w58 -> [w553]
        shift-right: [w563] -> w114
        shift-left: w111 -> [w561]
        shift-right: [w560] -> w110
        shift-left: w56 -> [w568]
        shift-right: [w522] -> _
        shift-left: w62 -> [w526]
        shift-right: [w521] -> _
        shift-left: w62 -> [w525]
        shift-right: [w520] -> _
        shift-left: w62 -> [w524]
        shift-right: [w519] -> _
        shift-left: w62 -> [w523]
        shift-right: [w515] -> _
        shift-left: w60 -> [w516]
        i -> [w567]
        stop <- w509 stop-if-true
        w547 = 0.0 ("t")
        w555 = T1 {"Integer Timestamp"=0, "Needle Voltage"=1.0, "Frequency"=0.0, "Width (ms) : 0.1 "=0.0, "Desired Amplitude (V)"=0.0, "Settings ID"="", "ID#"=0}  # Dust Source Controls
        w559 = T7 0 items=["no dialog", "OK message", "continue or stop message", "OK message + warnings", "continue/stop + warnings"] ("type of dialog (OK msg:1)")
        w558 = FALSE ("Blinking")
        # "On criteria - 0: Needle Voltage, 1: Desired Amplitude, 2: Width, 3: Frequency"
        # "Event structure to ramp up or ramp down (depending on what you want) pelletron controls"
        # "Throttling stuff"
        # "Output loop"
        n222 = property on="Actual Needle Output (V)" class="DigNum (strict)"("Blinking"=w558) -> ()  [unwired: 2 in, 2 out]
        n223 = property on="Actual output Amplitude (V)" class="DigNum (strict)"("Blinking"=w558) -> ()  [unwired: 2 in, 2 out]
        n224 = Reciprocal(x=w564) -> (1/x=w565:dbl)
        n225 = global read "throttle.vi" "Throttle"() -> (w527:bool)
        n226 = call-poly <userlib>:"Data Changed__ogtk.vi"("Boolean"=w527) -> ("Changed"=w529:bool)
        n227 = case shown="True" w529 {
          tunnel: w527 -> [_ w572]
          tunnel: "Frequency" -> [_ w571]
          frame False {
          }
          frame True {
            n228 = case shown="True" w572 {
              tunnel: w571 -> [_ w573]
              frame False {
              }
              frame True {
                "Freq. Before Throttle" <- w573
              }
            }
          }
        }
        n229 = global read "throttle from query.vi" "Throttle Q"() -> (w548:bool)
        n230 = Or(x=w548, y=w527) -> (x .or. y?=w549:bool)
        n231 = local read "Freq. Before Throttle"() -> (w530:dbl)
        n232 = Implies(1:w527, 2:w529) -> (0:w528:bool)
        n233 = Select(t=T6."Disabled and Grayed Out" ("Disabled"), s=w549, f=T6."Enabled" ("Disabled")) -> (s? t:f=w550:T6)
        n234 = property on="Frequency" class="DigNum (strict)"("DisabledEnum"=w550) -> ()  [unwired: 2 in, 2 out]
        n235 = Select(t=w547, s=w548, f="Frequency") -> (s? t:f=w545:dbl)
        n236 = Select(t=w547, s=w527, f=w545) -> (s? t:f=w541:dbl)
        n237 = Select(t=w541, s=w528, f=w530) -> (s? t:f=w531:dbl)
        n238 = Divide(x="Needle Voltage", y=1) -> (x/y=w557:dbl)
        n239 = call-poly <userlib>:"Data Changed__ogtk.vi"("DBL"=w531) -> ("Changed"=w546:bool)
        n240 = case shown="True" w546 {
          tunnel: w531 -> [_ w647]
          frame False {
          }
          frame True {
            n241 = property on="Frequency" class="DigNum (strict)"("Val(Sgnl)"=w647) -> ()  [unwired: 2 in, 2 out]
          }
        }
        n242 = Bundle By Name(cluster=w555, "Desired Amplitude (V)"="Desired Amplitude (V)", "Width (ms) : 0.1"="Width (ms) : 0.1", "Frequency"=w531, "Needle Voltage"="Needle Voltage") -> (→"output cluster":T1)
        n243 = Build Array("Needle Voltage", "Desired Amplitude (V)", "Width (ms) : 0.1", w531) -> (w540:dbl[])
        n244 = Greater?(x=w540, y=dbl[] [0.0, 0.0, 0.0, 0.0]) -> (0:w538:bool[])
        n245 = And Array Elements(Boolean array=w538) -> (logical AND=w517:bool)
        "On/Off" <- w517
        n246 = event shown="[5] \"Width (ms) : 0.1\": Value Change" {
          selector: _ -> [_ _ _ _ _ _]
          dyn-events: _ -> [_ _ _ _ _ _]
          timeout: 100 -> [_ _ _ _ _ _]
          tunnel: w566 -> [w657 w699 w763 w847 w906 w965]
          tunnel: w568 -> [w672 w694 w762 w832 w891 w950]
          tunnel: w531 -> [w652 w708 w764 w849 w908 w967]
          tunnel: "Width (ms) : 0.1" -> [w653 w709 w765 w850 w909 w968]
          tunnel: [w671 w693 w750 w830 w889 w948] -> w537
          tunnel: w561 -> [w670 w707 w757 w848 w907 w966]
          tunnel: "Desired Amplitude (V)" -> [w655 w691 w746 _ w888 w947]
          tunnel: w553 -> [w661 w704 w760 w844 w903 w962]
          tunnel: w565 -> [w660 w703 w761 w843 w902 w961]
          tunnel: [w664 w706 w758 w846 w905 w964] -> w563
          tunnel: [FALSE ("y") FALSE ("y") TRUE ("y") FALSE ("y") FALSE ("y") FALSE ("y")] -> w534
          tunnel: w557 -> [w659 _ w752 w840 w899 w958]
          tunnel: w526 -> [w651 w690 _ w828 w886 w945]
          tunnel: w525 -> [w650 w689 _ w829 w885 w944]
          tunnel: w524 -> [w649 w688 _ w827 w884 w946]
          tunnel: w523 -> [w648 w687 _ w826 w887 w943]
          tunnel: [w651 w681 w745 w828 w886 w945] -> w522
          tunnel: [w650 w689 w745 w820 w885 w944] -> w521
          tunnel: [w649 w688 w745 w827 w884 w937] -> w520
          tunnel: [w648 w687 w745 w826 w876 w943] -> w519
          event Timeout {
            w654 = FALSE ("Blinking")
            n247 = event-data() -> ()  [unwired: 1 in, 2 out]
            n248 = local write "Actual Needle Output (V)"(w659) -> ()
            n249 = local write "Actual output Amplitude (V)"(w655) -> ()
            n250 = call "Gen_Square_0to10V.vi"("sampling info"=w657, "error in (no error)"=w672, "Width (ms)"=w653, "amplitude"=w655, "frequency"=w652) -> ("error out"=w667:errorcluster, "signal out"=w656:waveform(dbl))  [unwired: 5 in]
            n251 = Initialize Array(w659, w661) -> (w662:dbl[])
            n252 = local write "Actual output width (ms)"(w653) -> ()
            n253 = local write "Actual output Frequency"(w652) -> ()
            n254 = local write "Output waveform"(w656) -> ()
            n255 = Bundle By Name("Y"=w662, "dt"=w660) -> (w658:waveform(dbl))  [unwired: 1 in]
            n256 = Merge Signals(w656, w658) -> (w665:dynamicdata)
            n257 = call-poly <vilib>:"DAQmx Write.vi"("task/channels in"=w670, "data"=w665, "error in"=w667) -> ("task out"=w669:refnum<k21>, "error out"=w666:errorcluster)  [unwired: 10 in, 1 out]
            n258 = First Call?() -> (First Call?: T/F=w668:bool)
            n259 = case shown="True" w668 {
              tunnel: [w673 w678] -> w671
              tunnel: [w674 w677] -> w664
              tunnel: w669 -> [w674 w676]
              tunnel: w666 -> [w673 w675]
              frame False {
              }
              frame True {
                n260 = call <vilib>:"DAQmx Start Task.vi"("task/channels in"=w676, "error in"=w675) -> ("task out"=w677:refnum<k21>, "error out"=w678:errorcluster)  [unwired: 12 in]
              }
            }
            n261 = property on="Actual output Amplitude (V)" class="DigNum (strict)"("Blinking"=w654) -> ()  [unwired: 2 in, 2 out]
            n262 = property on="Actual Needle Output (V)" class="DigNum (strict)"("Blinking"=w654) -> ()  [unwired: 2 in, 2 out]
            n263 = property on="Actual output width (ms)" class="DigNum (strict)"("Blinking"=w654) -> ()  [unwired: 2 in, 2 out]
            n264 = property on="Actual output Frequency" class="DigNum (strict)"("Blinking"=w654) -> ()  [unwired: 2 in, 2 out]
          }
          event "Needle Voltage": Value Change {
            (unwired) "needle" ("name (unnamed)")
            w700 = 0.05 ("y")
            n265 = event-data() -> ("NewVal"=w680:dbl)  [unwired: 1 in, 4 out]
            n266 = Greater?(x=w680, y=w690) -> (0:w702:bool)
            n267 = Subtract(x=w680, y=w690) -> (x-y=w696:dbl)
            n268 = Subtract(x=w690, y=w680) -> (x-y=w697:dbl)
            n269 = Greater?(x=w696, y=w697) -> (0:w698:bool)
            n270 = Select(t=w696, s=w698, f=w697) -> (s? t:f=w695:dbl)
            n271 = Divide(x=w695, y=w700) -> (x/y=w701:dbl)
            n272 = To Long Integer(number=w701) -> (32bit integer=w679:i32)
            n273 = for {
              N: w679 -> [_]
              tunnel: w700 -> [w740]
              tunnel: w690 -> [w739]
              tunnel: w703 -> [w737]
              tunnel: w704 -> [w736]
              tunnel: [w719] -> w692
              tunnel: w709 -> [w717]
              tunnel: w691 -> [w718]
              tunnel: w708 -> [w732]
              tunnel: w694 -> [w731]
              shift-right: [w735] -> w706
              shift-left: w707 -> [w730]
              tunnel: w702 -> [w724]
              tunnel: w699 -> [w723]
              tunnel: [w713] -> w682
              tunnel: [w711] -> w683
              i -> [w741]
              stop <- w711 stop-if-true
              n274 = local write "Actual output Amplitude (V)"(w718) -> ()
              n275 = call "Gen_Square_0to10V.vi"("sampling info"=w723, "error in (no error)"=w731, "Width (ms)"=w717, "amplitude"=w718, "frequency"=w732) -> ("error out"=w733:errorcluster, "signal out"=w720:waveform(dbl))  [unwired: 5 in]
              n276 = Increment(x=w741) -> (x+1=w742:i32)
              n277 = property on="Actual Needle Output (V)" class="DigNum (strict)"("Blinking"=TRUE) -> ()  [unwired: 2 in, 2 out]
              n278 = local write "Output waveform"(w720) -> ()
              n279 = Multiply(x=w740, y=w742) -> (x*y=w726:dbl)
              n280 = Negate(x=w726) -> (-x=w727:dbl)
              n281 = Select(t=w726, s=w724, f=w727) -> (s? t:f=w725:dbl)
              n282 = Add(x=w739, y=w725) -> (x+y=w722:dbl)
              n283 = Divide(x=w722, y=1.0) -> (x/y=w715:dbl)
              n284 = Less Than 0?(x=w715) -> (x < 0?=w716:bool)
              n285 = Select(t=0.0, s=w716, f=w715) -> (s? t:f=w713:dbl)
              n286 = local write "Actual Needle Output (V)"(w713) -> ()
              n287 = Initialize Array(w713, w736) -> (w738:dbl[])
              n288 = Bundle By Name("Y"=w738, "dt"=w737) -> (w728:waveform(dbl))  [unwired: 1 in]
              n289 = Merge Signals(w720, w728) -> (w734:dynamicdata)
              n290 = local read "Abort Change"() -> (w712:bool)
              n291 = local read "stop"() -> (w710:bool)
              n292 = call-poly <vilib>:"DAQmx Write.vi"("task/channels in"=w730, "data"=w734, "error in"=w733) -> ("task out"=w735:refnum<k21>, "error out"=w719:errorcluster)  [unwired: 10 in, 1 out]
              n293 = Or(x=w712, y=w710) -> (x .or. y?=w711:bool)
              n294 = case shown="True" w711 {
                tunnel: w713 -> [_ w743]
                frame False {
                }
                frame True {
                  n295 = local write "Needle Voltage"(w743) -> ()
                }
              }
            }
            n296 = Equal To 0?(x=w679) -> (x = 0?=w685:bool)
            n297 = Not(x=w683) -> (.not. x?=w686:bool)
            n298 = Merge Errors(w692) -> (w693:errorcluster)
            n299 = Or(x=w686, y=w685) -> (x .or. y?=w684:bool)
            n300 = Select(t=w680, s=w684, f=w682) -> (s? t:f=w681:dbl)
          }
          event "stop": Value Change {
            w745 = 0.0 ("Width (ms) : 3.5")
            w749 = TRUE ("Blinking")
            n301 = event-data() -> ()  [unwired: 1 in, 1 out]
            n302 = property on="Actual Needle Output (V)" class="DigNum (strict)"("Blinking"=w749) -> ()  [unwired: 2 in, 2 out]
            n303 = property on="Actual output Amplitude (V)" class="DigNum (strict)"("Blinking"=w749) -> ()  [unwired: 2 in, 2 out]
            n304 = Multiply(x=w752, y=20.0 ("x")) -> (x*y=w754:dbl)
            n305 = Multiply(x=20.0, y=w746) -> (x*y=w744:dbl)
            n306 = Greater?(x=w754, y=w744) -> (0:w753:bool)
            n307 = Select(t=w754, s=w753, f=w744) -> (s? t:f=w747:dbl)
            n308 = Increment(x=w747) -> (x+1=w748:dbl)
            n309 = for {
              N: w748 -> [w773]
              tunnel: w765 -> [w786]
              tunnel: w764 -> [w785]
              tunnel: w763 -> [w779]
              tunnel: w746 -> [w787]
              tunnel: w760 -> [w777]
              tunnel: w761 -> [w776]
              tunnel: [w776] -> _ mode=indexing
              shift-right: [w781] -> w751
              shift-left: w762 -> [w780]
              tunnel: w752 -> [w769]
              tunnel: w757 -> [w783]
              tunnel: [w784] -> w758
              i -> [w775]
              n310 = Subtract(x=w773, y=1) -> (x-y=w772:i32)
              n311 = Wait (ms)(milliseconds to wait=u32 250) -> ()  [unwired: 1 out]
              n312 = Equal?(x=w772, y=w775) -> (x = y?=w774:bool)
              n313 = case shown="True" w774 {
                tunnel: w787 -> [w810 _]
                tunnel: w786 -> [w809 _]
                tunnel: w785 -> [w808 _]
                tunnel: [w807 w816] -> w782
                tunnel: w780 -> [w806 w816]
                tunnel: w779 -> [w802 _]
                tunnel: [w801 w817] -> w778
                tunnel: w773 -> [w798 _]
                tunnel: w777 -> [w794 w812]
                tunnel: w776 -> [w796 w814]
                tunnel: w775 -> [w788 _]
                tunnel: w769 -> [w797 _]
                tunnel: [w790 w815] -> w768
                frame False {
                  n314 = Divide(x=w797, y=w798) -> (x/y=w800:dbl)
                  n315 = Divide(x=w810, y=w798) -> (x/y=w805:dbl)
                  n316 = Multiply(x=w800, y=w788) -> (x*y=w799:dbl)
                  n317 = Multiply(x=w805, y=w788) -> (x*y=w804:dbl)
                  n318 = Subtract(x=w797, y=w799) -> (x-y=w791:dbl)
                  n319 = Subtract(x=w810, y=w804) -> (x-y=w803:dbl)
                  n320 = local write "Actual output Amplitude (V)"(w803) -> ()
                  n321 = call "Gen_Square_0to10V.vi"("sampling info"=w802, "error in (no error)"=w806, "Width (ms)"=w809, "amplitude"=w803, "frequency"=w808) -> ("error out"=w807:errorcluster, "signal out"=w790:waveform(dbl))  [unwired: 5 in]
                  n322 = Divide(x=w791, y=1.0) -> (x/y=w792:dbl)
                  n323 = local write "Actual Needle Output (V)"(w792) -> ()
                  n324 = Initialize Array(w792, w794) -> (w795:dbl[])
                  n325 = Bundle By Name("Y"=w795, "dt"=w796) -> (w789:waveform(dbl))  [unwired: 1 in]
                  n326 = Merge Signals(w790, w789) -> (w801:dynamicdata)
                }
                frame True {
                  w813 = 0.0 ("element")
                  n327 = local write "Actual Needle Output (V)"(w813) -> ()
                  n328 = local write "Needle Voltage"(w813) -> ()
                  n329 = local write "Desired Amplitude (V)"(w813) -> ()
                  n330 = local write "Actual output Amplitude (V)"(w813) -> ()
                  n331 = Initialize Array(w813, w812) -> (w811:dbl[])
                  n332 = Bundle By Name("Y"=w811, "dt"=w814) -> (w815:waveform(dbl))  [unwired: 1 in]
                  n333 = Merge Signals(w815, w815) -> (w817:dynamicdata)
                }
              }
              n334 = local write "Output waveform"(w768) -> ()
              n335 = call-poly <vilib>:"DAQmx Write.vi"("task/channels in"=w783, "data"=w778, "error in"=w782) -> ("task out"=w784:refnum<k21>, "error out"=w781:errorcluster)  [unwired: 10 in, 1 out]
            }
            n336 = flat-sequence {
              tunnel: w751 -> [w767]
              tunnel: [w767] -> w750
              frame #0 {
                w766 = TRUE ("Finished")
                n337 = local write "stop"(w766) -> ()
                "Finished" <- w766
              }
            }
          }
          event "Desired Amplitude (V)": Value Change {
            w837 = 0.05 ("y")
            n338 = event-data() -> ("NewVal"=w819:dbl)  [unwired: 1 in, 1 out]
            n339 = local write "Actual Needle Output (V)"(w840) -> ()
            n340 = Greater?(x=w819, y=w829) -> (0:w839:bool)
            n341 = Subtract(x=w819, y=w829) -> (x-y=w835:dbl)
            n342 = Subtract(x=w829, y=w819) -> (x-y=w833:dbl)
            n343 = Initialize Array(w840, w844) -> (w842:dbl[])
            n344 = Greater?(x=w835, y=w833) -> (0:w836:bool)
            n345 = Bundle By Name("Y"=w842, "dt"=w843) -> (w841:waveform(dbl))  [unwired: 1 in]
            n346 = Select(t=w835, s=w836, f=w833) -> (s? t:f=w834:dbl)
            n347 = Quotient & Remainder(x=w834, y=w837) -> (floor(x/y)=w838:dbl)  [unwired: 1 out]
            n348 = To Long Integer(number=w838) -> (32bit integer=w818:i32)
            n349 = for {
              N: w818 -> [_]
              tunnel: w850 -> [w873]
              tunnel: w849 -> [w872]
              tunnel: w829 -> [w870]
              tunnel: w832 -> [w869]
              tunnel: [w867] -> w831
              tunnel: w847 -> [w865]
              tunnel: w837 -> [w862]
              tunnel: w841 -> [w860]
              shift-right: [w866] -> w846
              shift-left: w848 -> [w868]
              tunnel: w839 -> [w856]
              tunnel: [w854] -> w821
              tunnel: [w852] -> w822
              i -> [w871]
              stop <- w852 stop-if-true
              n350 = Increment(x=w871) -> (x+1=w864:i32)
              n351 = property on="Actual output Amplitude (V)" class="DigNum (strict)"("Blinking"=TRUE) -> ()  [unwired: 2 in, 2 out]
              n352 = Multiply(x=w862, y=w864) -> (x*y=w857:dbl)
              n353 = Negate(x=w857) -> (-x=w859:dbl)
              n354 = Select(t=w857, s=w856, f=w859) -> (s? t:f=w858:dbl)
              n355 = Add(x=w870, y=w858) -> (x+y=w854:dbl)
              n356 = local write "Actual output Amplitude (V)"(w854) -> ()
              n357 = call "Gen_Square_0to10V.vi"("sampling info"=w865, "error in (no error)"=w869, "Width (ms)"=w873, "amplitude"=w854, "frequency"=w872) -> ("error out"=w874:errorcluster, "signal out"=w855:waveform(dbl))  [unwired: 5 in]
              n358 = local write "Output waveform"(w855) -> ()
              n359 = Merge Signals(w855, w860) -> (w861:dynamicdata)
              n360 = call-poly <vilib>:"DAQmx Write.vi"("task/channels in"=w868, "data"=w861, "error in"=w874) -> ("task out"=w866:refnum<k21>, "error out"=w867:errorcluster)  [unwired: 10 in, 1 out]
              n361 = local read "Abort Change"() -> (w853:bool)
              n362 = local read "stop"() -> (w851:bool)
              n363 = Or(x=w853, y=w851) -> (x .or. y?=w852:bool)
              n364 = case shown="True" w852 {
                tunnel: w854 -> [_ w875]
                frame False {
                }
                frame True {
                  n365 = local write "Desired Amplitude (V)"(w875) -> ()
                }
              }
            }
            n366 = Equal To 0?(x=w818) -> (x = 0?=w824:bool)
            n367 = Not(x=w822) -> (.not. x?=w825:bool)
            n368 = Merge Errors(w831) -> (w830:errorcluster)
            n369 = Or(x=w825, y=w824) -> (x .or. y?=w823:bool)
            n370 = Select(t=w819, s=w823, f=w821) -> (s? t:f=w820:dbl)
          }
          event "Frequency": Value Change {
            w896 = 0.5 ("y")
            n371 = event-data() -> ("NewVal"=w878:dbl)  [unwired: 1 in, 1 out]
            n372 = local write "Actual Needle Output (V)"(w899) -> ()
            n373 = Greater?(x=w878, y=w887) -> (0:w898:bool)
            n374 = Subtract(x=w878, y=w887) -> (x-y=w894:dbl)
            n375 = Subtract(x=w887, y=w878) -> (x-y=w892:dbl)
            n376 = Initialize Array(w899, w903) -> (w901:dbl[])
            n377 = Greater?(x=w894, y=w892) -> (0:w895:bool)
            n378 = Bundle By Name("Y"=w901, "dt"=w902) -> (w900:waveform(dbl))  [unwired: 1 in]
            n379 = Select(t=w894, s=w895, f=w892) -> (s? t:f=w893:dbl)
            n380 = Quotient & Remainder(x=w893, y=w896) -> (floor(x/y)=w897:dbl)  [unwired: 1 out]
            n381 = To Long Integer(number=w897) -> (32bit integer=w877:i32)
            n382 = for {
              N: w877 -> [_]
              tunnel: w909 -> [w932]
              tunnel: w908 -> [_]
              tunnel: w887 -> [w930]
              tunnel: w891 -> [w929]
              tunnel: [w927] -> w890
              tunnel: w906 -> [w925]
              tunnel: w896 -> [w923]
              tunnel: w900 -> [w921]
              shift-right: [w926] -> w905
              shift-left: w907 -> [w928]
              tunnel: w898 -> [w917]
              tunnel: w888 -> [w914]
              tunnel: [w913] -> w879
              tunnel: [w911] -> w880
              i -> [w931]
              stop <- w911 stop-if-true
              n383 = Increment(x=w931) -> (x+1=w924:i32)
              n384 = Multiply(x=w923, y=w924) -> (x*y=w918:dbl)
              n385 = property on="Actual output Frequency" class="DigNum (strict)"("Blinking"=TRUE) -> ()  [unwired: 2 in, 2 out]
              n386 = Negate(x=w918) -> (-x=w920:dbl)
              n387 = Select(t=w918, s=w917, f=w920) -> (s? t:f=w919:dbl)
              n388 = Add(x=w930, y=w919) -> (x+y=w913:dbl)
              n389 = call "Gen_Square_0to10V.vi"("sampling info"=w925, "error in (no error)"=w929, "Width (ms)"=w932, "amplitude"=w914, "frequency"=w913) -> ("error out"=w933:errorcluster, "signal out"=w916:waveform(dbl))  [unwired: 5 in]
              n390 = local write "Actual output Frequency"(w913) -> ()
              n391 = local write "Output waveform"(w916) -> ()
              n392 = Merge Signals(w916, w921) -> (w922:dynamicdata)
              n393 = local read "Abort Change"() -> (w912:bool)
              n394 = call-poly <vilib>:"DAQmx Write.vi"("task/channels in"=w928, "data"=w922, "error in"=w933) -> ("task out"=w926:refnum<k21>, "error out"=w927:errorcluster)  [unwired: 10 in, 1 out]
              n395 = local read "stop"() -> (w910:bool)
              n396 = Or(x=w912, y=w910) -> (x .or. y?=w911:bool)
              n397 = case shown="True" w911 {
                tunnel: w913 -> [_ w934]
                frame False {
                }
                frame True {
                  n398 = local write "Frequency"(w934) -> ()
                }
              }
            }
            n399 = Equal To 0?(x=w877) -> (x = 0?=w882:bool)
            n400 = Not(x=w880) -> (.not. x?=w883:bool)
            n401 = Merge Errors(w890) -> (w889:errorcluster)
            n402 = Or(x=w883, y=w882) -> (x .or. y?=w881:bool)
            n403 = Select(t=w878, s=w881, f=w879) -> (s? t:f=w876:dbl)
          }
          event "Width (ms) : 0.1": Value Change {
            w955 = 0.1 ("y")
            n404 = event-data() -> ("NewVal"=w935:dbl)  [unwired: 1 in, 1 out]
            n405 = local write "Actual Needle Output (V)"(w958) -> ()
            n406 = Greater?(x=w935, y=w946) -> (0:w957:bool)
            n407 = Subtract(x=w935, y=w946) -> (x-y=w953:dbl)
            n408 = Subtract(x=w946, y=w935) -> (x-y=w951:dbl)
            n409 = Initialize Array(w958, w962) -> (w960:dbl[])
            n410 = Greater?(x=w953, y=w951) -> (0:w954:bool)
            n411 = Bundle By Name("Y"=w960, "dt"=w961) -> (w959:waveform(dbl))  [unwired: 1 in]
            n412 = Select(t=w953, s=w954, f=w951) -> (s? t:f=w952:dbl)
            n413 = Quotient & Remainder(x=w952, y=w955) -> (floor(x/y)=w956:dbl)  [unwired: 1 out]
            n414 = To Long Integer(number=w956) -> (32bit integer=w939:i32)
            n415 = for {
              N: w939 -> [_]
              tunnel: w968 -> [_]
              tunnel: w967 -> [w991]
              tunnel: w946 -> [w989]
              tunnel: w950 -> [w988]
              tunnel: [w986] -> w949
              tunnel: w965 -> [w984]
              tunnel: w955 -> [w982]
              tunnel: w959 -> [w980]
              shift-right: [w985] -> w964
              shift-left: w966 -> [w987]
              tunnel: w957 -> [w976]
              tunnel: w947 -> [w974]
              tunnel: [w972] -> w936
              tunnel: [w970] -> w942
              i -> [w990]
              stop <- w970 stop-if-true
              n416 = Increment(x=w990) -> (x+1=w983:i32)
              n417 = Multiply(x=w982, y=w983) -> (x*y=w977:dbl)
              n418 = property on="Actual output width (ms)" class="DigNum (strict)"("Blinking"=TRUE) -> ()  [unwired: 2 in, 2 out]
              n419 = Negate(x=w977) -> (-x=w979:dbl)
              n420 = Select(t=w977, s=w976, f=w979) -> (s? t:f=w978:dbl)
              n421 = Add(x=w989, y=w978) -> (x+y=w972:dbl)
              n422 = call "Gen_Square_0to10V.vi"("sampling info"=w984, "error in (no error)"=w988, "Width (ms)"=w972, "amplitude"=w974, "frequency"=w991) -> ("error out"=w992:errorcluster, "signal out"=w975:waveform(dbl))  [unwired: 5 in]
              n423 = local write "Actual output width (ms)"(w972) -> ()
              n424 = local write "Output waveform"(w975) -> ()
              n425 = Merge Signals(w975, w980) -> (w981:dynamicdata)
              n426 = local read "Abort Change"() -> (w971:bool)
              n427 = call-poly <vilib>:"DAQmx Write.vi"("task/channels in"=w987, "data"=w981, "error in"=w992) -> ("task out"=w985:refnum<k21>, "error out"=w986:errorcluster)  [unwired: 10 in, 1 out]
              n428 = local read "stop"() -> (w969:bool)
              n429 = Or(x=w969, y=w971) -> (x .or. y?=w970:bool)
              n430 = case shown="True" w970 {
                tunnel: w972 -> [_ w993]
                frame False {
                }
                frame True {
                  n431 = local write "Width (ms) : 0.1"(w993) -> ()
                }
              }
            }
            n432 = Equal To 0?(x=w939) -> (x = 0?=w940:bool)
            n433 = Not(x=w942) -> (.not. x?=w941:bool)
            n434 = Or(x=w941, y=w940) -> (x .or. y?=w938:bool)
            n435 = Merge Errors(w949) -> (w948:errorcluster)
            n436 = Select(t=w935, s=w938, f=w936) -> (s? t:f=w937:dbl)
          }
        }
        n437 = call-poly <userlib>:"Data Changed__ogtk.vi"("Boolean"=w517) -> ("Changed"=w518:bool)
        n438 = And(x=w534, y=w517) -> (x .and. y?=w533:bool)
        n439 = Or(x=w533, y=w518) -> (x .or. y?=w535:bool)
        n440 = local read "Testing"() -> (w513:bool)
        n441 = case shown="True" w535 {
          tunnel: w517 -> [_ w578]
          tunnel: w537 -> [w575 w583]
          tunnel: [w575 w582] -> w536
          tunnel: w533 -> [_ w577]
          tunnel: w516 -> [w574 w581]
          tunnel: [w574 w580] -> w515
          frame False {
          }
          frame True {
            n442 = Select(t=FALSE, s=w577, f=w578) -> (s? t:f=w579:bool)
            n443 = case shown="False" w579 {
              tunnel: w583 -> [w605 w646]
              tunnel: [w602 w646] -> w582
              tunnel: w581 -> [w584 _]
              tunnel: [w584 w644] -> w580
              frame False {
                n444 = Get Date/Time In Seconds() -> (seconds since 1Jan1904=w608:timestamp)
                n445 = call "timestamp_conversion.vi"("error in (no error)"=w605, "Time Stamp"=w608) -> ("error out"=w606:errorcluster, "Integer Time"=w585:i64)  [unwired: 7 in]
                n446 = call "connect in.vi"("error in (no error)"=w606) -> ("error out"=w600:errorcluster, "Database Connection"=w601:T4)  [unwired: 6 in, 1 out]
                n447 = call-poly <vilib>:"DB Tools Execute Query.vi"("error in (no error)"=w600, "SQL query"="SELECT id_experiment_settings\nFROM experiment_settings_small\nORDER BY integer_timestamp DESC\nLIMIT 1; ", "connection reference"=w601) -> ("error out"=w598:errorcluster, "recordset reference"=w599:T5)  [unwired: 5 in]
                n448 = call-poly <vilib>:"DB Tools Fetch Recordset Data.vi"("error in (no error)"=w598, "recordset reference"=w599) -> ("error out"=w587:errorcluster, "recordset data"=w593:variant[][], "recordset reference out"=w597:T5)  [unwired: 3 in]
                n449 = Index Array(array=w593, index (row)=0, index (col)=0 ("disabled index (col)")) -> (element=w590:variant)
                n450 = xnode "Database Variant To Data"("database variant"=w590, "error in (no error)"=w587, "type"=0) -> ("data"=w588:i32, "error out"=w586:errorcluster)
                n451 = call-poly <vilib>:"DB Tools Free Object.vi"("error in (no error)"=w586, "recordset reference"=w597) -> ("error out"=w595:errorcluster, "connection reference"=w596:T4)  [unwired: 8 in]
                n452 = Bundle("Integer Time"=w584, "Integer Time"=w585, "data"=w588) -> (w607:T8)  [unwired: 1 in]
                n453 = call <vilib>:"DB Tools Insert Data.vi"("create table? (F)"=FALSE, "data"=w607, "error in (no error)"=w595, "table"="run_times_small", "connection reference"=w596) -> ("error out"=w603:errorcluster, "connection reference out"=w610:T4)  [unwired: 5 in]
                n454 = call "connect out.vi"("error in (no error)"=w600, "connection reference"=w610) -> ("error out"=w604:errorcluster)  [unwired: 9 in]
                n455 = Merge Errors(w603, w604) -> (w602:errorcluster)
              }
              frame True {
                n456 = Get Date/Time In Seconds() -> (seconds since 1Jan1904=w645:timestamp)
                n457 = call "timestamp_conversion.vi"("Time Stamp"=w645) -> ("Integer Time"=w644:i64)  [unwired: 8 in, 1 out]
              }
            }
          }
        }
        n458 = Unbundle By Name(w536) -> ("status"=w512:bool)
        n459 = call <vilib>:"Simple Error Handler.vi"("type of dialog (OK msg:1)"=w559, "error in (no error)"=w536) -> ("error?"=w514:bool, "error out"=w560:errorcluster)  [unwired: 3 in, 3 out]
        n460 = Not(x=w513) -> (.not. x?=w507:bool)
        n461 = case shown="False" w513 {
          tunnel: w514 -> [w569 w570]
          tunnel: [w569 w570] -> w510
          frame False {
            n462 = property on="error?" class="Bool (strict)"("Val(Sgnl)"=w569) -> ()  [unwired: 2 in, 2 out]
          }
          frame True {
          }
        }
        n463 = And(x=w507, y=w512) -> (x .and. y?=w511:bool)
        n464 = Or(x=w511, y=w534) -> (x .or. y?=w509:bool)
        n465 = And(x=w507, y=w510) -> (x .and. y?=→"error?":bool)
        "Execution Number:" <- w567
      }
      n466 = call <vilib>:"DAQmx Clear Task.vi"("task in"=w63, "error in"=w78) -> ("error out"=w77:errorcluster)  [unwired: 13 in]
      n467 = call <vilib>:"DAQmx Stop Task.vi"("task/channels in"=w100, "error in"=w99) -> ("task out"=w96:refnum<k21>, "error out"=w95:errorcluster)  [unwired: 12 in]
      n468 = call <vilib>:"DAQmx Stop Task.vi"("task/channels in"=w98, "error in"=w97) -> ("task out"=w94:refnum<k21>, "error out"=w93:errorcluster)  [unwired: 12 in]
      n469 = call <vilib>:"DAQmx Clear Task.vi"("task in"=w96, "error in"=w95) -> ("error out"=w88:errorcluster)  [unwired: 13 in]
      n470 = call <vilib>:"DAQmx Clear Task.vi"("task in"=w94, "error in"=w93) -> ("error out"=w87:errorcluster)  [unwired: 13 in]
      n471 = Merge Errors(w88, w87, w59) -> (w85:errorcluster)
      n472 = call <vilib>:"DAQmx Clear Task.vi"("task in"=w114, "error in"=w110) -> ("error out"=w113:errorcluster)  [unwired: 13 in]
      n473 = call <vilib>:"Simple Error Handler.vi"("type of dialog (OK msg:1)"=w125, "error in (no error)"=w113) -> ("error out"=w112:errorcluster)  [unwired: 3 in, 4 out]
      n474 = Merge Errors(w112, w85, w77, w86) -> (w108:errorcluster)
      n475 = while {
        tunnel: [w292] -> w107
        tunnel: w108 -> [w292]
        stop <- w293 stop-if-true
        # "Loop to ask if the batteries are off"
        n476 = Two Button Dialog(message="Have you turned off the High voltage?", 1:"No, thank you for reminding me! I'll go do that right now!" ("button name (\"OK\")"), 2:"Yes, of course I have." ("T button name (\"OK\")")) -> (T button?=w293:bool)
      }
    }
    frame Error {
    }
  }
  "error out" <- w52
